vi "Mouse Move.vi"(8 "error in (no error)":errorcluster, 10 "Point":T1, 11 "Geometric Object in":refnum<class "Graphics Object.lvclass">) -> (0 "error out":errorcluster, 3 "Geometric Object out":refnum<class "Graphics Object.lvclass">)   [LabVIEW 2018, in "Graphics Object.lvclass"]
doc: "A method for specifying how a graphics object reacts on a mouse move event."
uses:
  Graphics Object.lvclass
  <vilib>/Utility/miscctls.llb/LVPoint32TypeDef.ctl
panel:
  # "expressionflow.com"
  # "Copyright (c) 2008 Tomi Maila. All rights reserved."
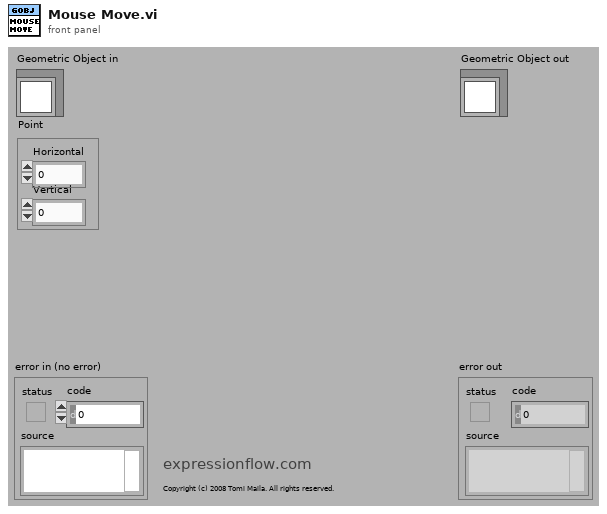
[diagram p1: front panel]
types:
  T1 = typedef "LVPoint32TypeDef.ctl" = cluster{"Horizontal":i32, "Vertical":i32}
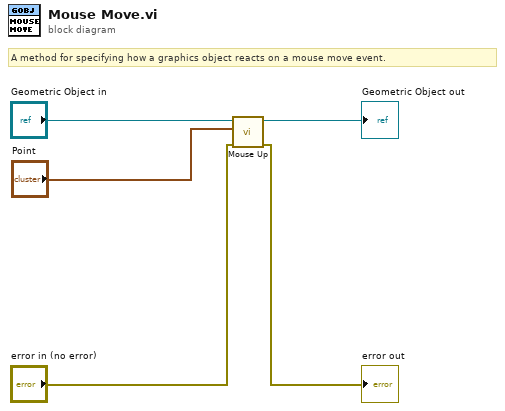
[diagram p0: block diagram]
diagram:
  # "A method for specifying how a graphics object reacts on a mouse move event."
  n1 = call-dynamic "Mouse Up.vi"("error in (no error)"="error in (no error)", "Point"="Point", "Geometric Object in"="Geometric Object in") -> ("error out"=→"error out":errorcluster, "Geometric Object out"=→"Geometric Object out":refnum<class "Graphics Object.lvclass">)  [unwired: 7 in]
